vi "Publish Element.vi"(6 "Synchronous":bool, 8 "Timeout mS (-1)":i32, 9 "element":T1, 11 "Channel Data In":T2) -> (1 "Closed":bool, 2 "Timeout":bool)   [LabVIEW 2022 SP3, in "Flex.lvlib"]
uses:
  Flex.lvlib
  Channel Data.ctl
  Element Info.ctl
  Element.ctl
  Event Data.ctl
  Writer Data.ctl
  Queue Data.ctl
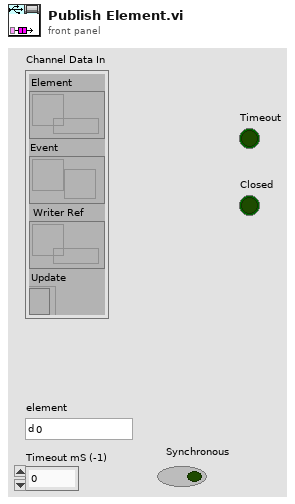
[diagram p1: front panel]
types:
  T1 = typedef "Flex.lvlib/Element.ctl" = dbl
  T2 = typedef "Flex.lvlib/Channel Data.ctl" = cluster{"Element":refnum<data-value>, "Event":refnum<user-event>, "Writer Ref":refnum<data-value>, "Update":refnum<k4>}
  T3 = typedef "Flex.lvlib/Writer Data.ctl" = cluster{"Lossless":refnum<queue>[], "Events":bool, "Lossy":bool}
  T4 = typedef "Flex.lvlib/Queue Data.ctl" = cluster{"element":T1, "Flags":u8}
  T5 = typedef "Flex.lvlib/Event Data.ctl" = cluster{"Value":T1, "Closed":bool}
  T6 = typedef "Flex.lvlib/Element Info.ctl" = cluster{"Value":T1, "Updated":timestamp, "Sequence":u32, "Paused":bool}
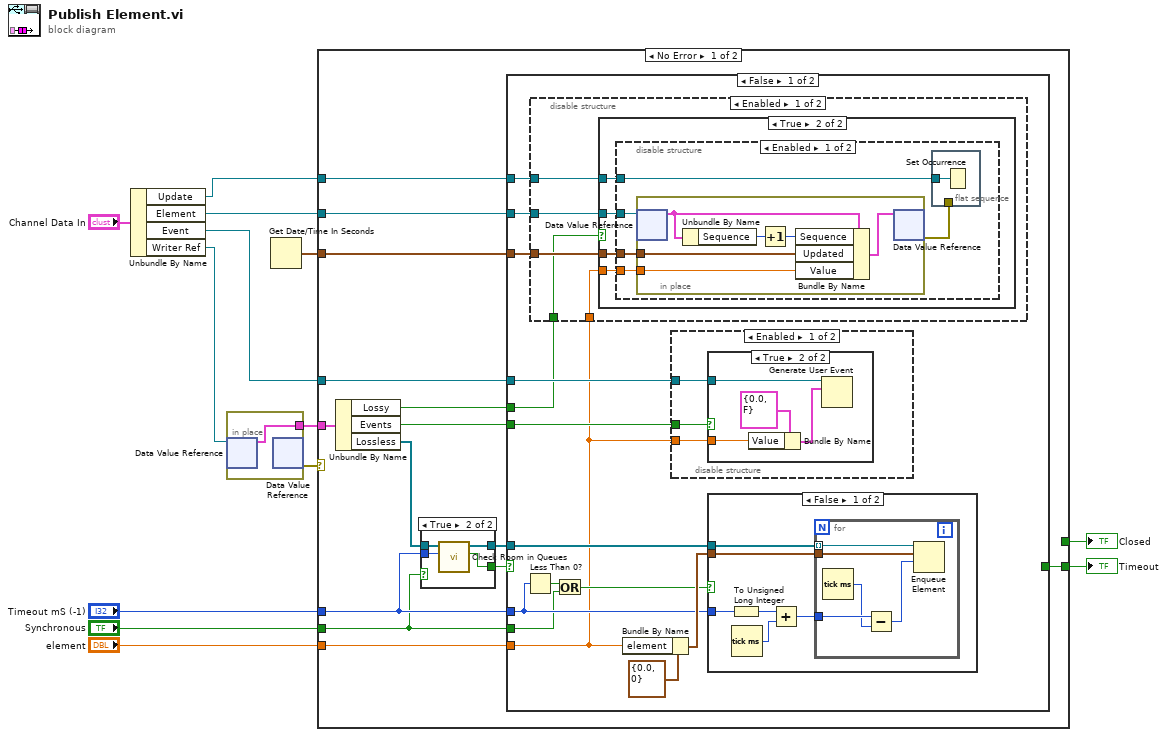
[diagram p0: block diagram]
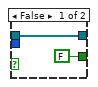
[diagram p2: hidden frame]
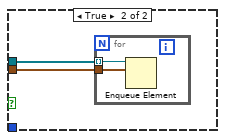
[diagram p8: hidden frame]
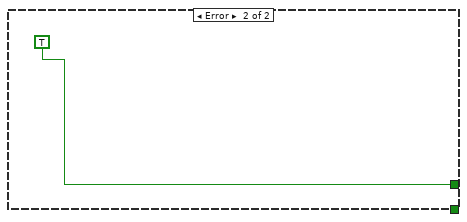
[diagram p10: hidden frame]
diagram:
  n1 = Unbundle By Name("Channel Data In") -> ("Update"=w1:refnum<k4>, "Element"=w2:refnum<data-value>, "Event"=w3:refnum<user-event>, "Writer Ref"=w12:refnum<data-value>)
  n2 = in-place {
    in-place-border: [w14] -> w11
    n3 = in-place-dvr #1(w12) -> (w14:T3)  [unwired: 1 out]
    n4 = in-place-dvr #1() -> (w8:errorcluster)  [unwired: 1 in, 1 out]
  }
  n5 = Get Date/Time In Seconds() -> (seconds since 1Jan1904=w6:timestamp)
  n6 = case shown="No Error" w8 {
    tunnel: w11 -> [w21 _]
    tunnel: "Timeout mS (-1)" -> [w22 _]
    tunnel: "element" -> [w28 _]
    tunnel: [_ TRUE] -> w7
    tunnel: w6 -> [w27 _]
    tunnel: [w24 _] -> w5
    tunnel: w3 -> [w23 _]
    tunnel: "Synchronous" -> [w16 _]
    tunnel: w2 -> [w18 _]
    tunnel: w1 -> [w15 _]
    frame No Error {
      n7 = Unbundle By Name(w21) -> ("Lossy"=w17:bool, "Events"=w19:bool, "Lossless"=w20:refnum<queue>[])
      n8 = case shown="True" w16 {
        tunnel: w22 -> [_ w34]
        tunnel: [w29 w33] -> w26
        tunnel: [FALSE ("Timeout") w32] -> w25
        tunnel: w20 -> [w29 w31]
        frame False {
        }
        frame True {
          n9 = call "Check Room in Queues.vi"("Timeout mS"=w34, "Queues In"=w31) -> ("Timeout"=w32:bool, "Queues"=w33:refnum<queue>[])  [unwired: 8 in]
        }
      }
      n10 = case shown="False" w25 {
        selector: w25 -> [_ w92]
        tunnel: w28 -> [w37 _]
        tunnel: w27 -> [w38 _]
        tunnel: w26 -> [w48 _]
        tunnel: [_ w92] -> w24
        tunnel: w23 -> [w47 _]
        tunnel: w16 -> [w42 _]
        tunnel: w22 -> [w44 _]
        tunnel: w19 -> [w40 _]
        tunnel: w18 -> [w39 _]
        tunnel: w17 -> [w36 _]
        tunnel: w15 -> [w35 _]
        frame False {
          n11 = Less Than 0?(x=w44) -> (x < 0?=w43:bool)
          n12 = disable-structure shown="Enabled" {
            disable-tunnel: w39 -> [w53 _]
            disable-tunnel: w38 -> [w52 _]
            disable-tunnel: w37 -> [w51 _]
            disable-tunnel: w36 -> [w50 _]
            disable-tunnel: w35 -> [w49 _]
            frame Enabled {
              n13 = case shown="True" w50 {
                tunnel: w53 -> [_ w57]
                tunnel: w52 -> [_ w56]
                tunnel: w51 -> [_ w55]
                tunnel: w49 -> [_ w54]
                frame False {
                }
                frame True {
                  n14 = disable-structure shown="Enabled" {
                    disable-tunnel: w57 -> [w62 _]
                    disable-tunnel: w56 -> [w61 _]
                    disable-tunnel: w55 -> [w60 _]
                    disable-tunnel: w54 -> [w58 _]
                    frame Enabled {
                      n15 = in-place {
                        in-place-border: w61 -> [w69]
                        in-place-border: w60 -> [w67]
                        n16 = in-place-dvr #2(w62) -> (w68:T6)  [unwired: 1 out]
                        n17 = Unbundle By Name(w68) -> ("Sequence"=w66:u32)
                        n18 = Increment(x=w66) -> (x+1=w65:u32)
                        n19 = Bundle By Name(cluster=w68, "Sequence"=w65, "Updated"=w69, "Value"=w67) -> (w64:T6)
                        n20 = in-place-dvr #2(w64) -> (w59:errorcluster)  [unwired: 1 out]
                      }
                      n21 = flat-sequence {
                        tunnel: w59 -> [_]
                        tunnel: w58 -> [w63]
                        frame #0 {
                          n22 = Set Occurrence(w63) -> ()
                        }
                      }
                    }
                    frame Disabled {
                    }
                  }
                }
              }
            }
            frame Disabled {
            }
          }
          n23 = Or(x=w43, y=w42) -> (x .or. y?=w41:bool)
          n24 = Bundle By Name(cluster=T4 {"element"=0.0, "Flags"=0} ("Queue Data"), "element"=w37) -> (w45:T4)
          n25 = disable-structure shown="Enabled" {
            disable-tunnel: w47 -> [w72 _]
            disable-tunnel: w40 -> [w71 _]
            disable-tunnel: w37 -> [w70 _]
            frame Enabled {
              n26 = case shown="True" w71 {
                tunnel: w72 -> [_ w76]
                tunnel: w70 -> [_ w75]
                frame False {
                }
                frame True {
                  n27 = Bundle By Name(cluster=T5 {"Value"=0.0, "Closed"=FALSE} ("event data"), "Value"=w75) -> (w73:T5)
                  n28 = Generate User Event(user event=w76, event data cluster=w73) -> ()  [unwired: 2 in, 2 out]
                }
              }
            }
            frame Disabled {
            }
          }
          n29 = case shown="False" w41 {
            tunnel: w48 -> [w82 w89]
            tunnel: w45 -> [w81 w88]
            tunnel: w44 -> [w79 _]
            frame False {
              n30 = To Unsigned Long Integer(number=w79) -> (unsigned 32bit integer=w77:u32)
              n31 = Tick Count (ms)() -> (millisecond timer value=w80:u32)
              n32 = Add(x=w77, y=w80) -> (x+y=w78:u32)
              n33 = for {
                tunnel: w82 -> [w87] mode=indexing
                tunnel: w81 -> [w86]
                tunnel: w78 -> [w85]
                n34 = Tick Count (ms)() -> (millisecond timer value=w84:u32)
                n35 = Subtract(x=w85, y=w84) -> (x-y=w83:i32)
                n36 = Enqueue Element(queue=w87, element=w86, timeout in ms (-1)=w83) -> ()  [unwired: 1 in, 3 out]
              }
            }
            frame True {
              n37 = for {
                tunnel: w89 -> [w91] mode=indexing
                tunnel: w88 -> [w90]
                n38 = Enqueue Element(queue=w91, element=w90) -> ()  [unwired: 2 in, 3 out]
              }
            }
          }
        }
        frame True {
        }
      }
    }
    frame Error {
    }
  }
  "Timeout" <- w5
  "Closed" <- w7
